vi "自动添加所有参数数据.vi"(8 "error in (no error)":errorcluster, 11 "数据类别":enum16{"水样数据", "日质控数据"}(ring)) -> (0 "错误输出":errorcluster)   [LabVIEW 2016, in "数据查询.lvlib"]
uses:
  <vilib>/Utility/config.llb/Read Key (Boolean).vi
  <vilib>/Utility/config.llb/Write Key (Boolean).vi
  <vilib>/Utility/config.llb/Read Key (String).vi
  <vilib>/Utility/config.llb/Write Key (String).vi
  <vilib>/Utility/config.llb/NI_LVConfig.lvlib
panel:
  out "数组":timestamp[](array[timestamp])
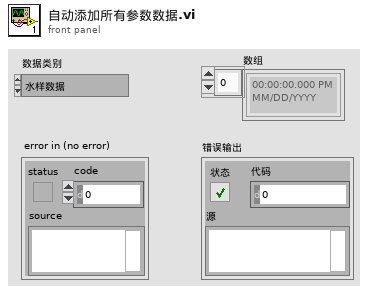
[diagram p1: front panel]
types:
  T1 = typedef "NI_LVConfig.lvlib/Config Data RefNum.ctl" = refnum<k1>
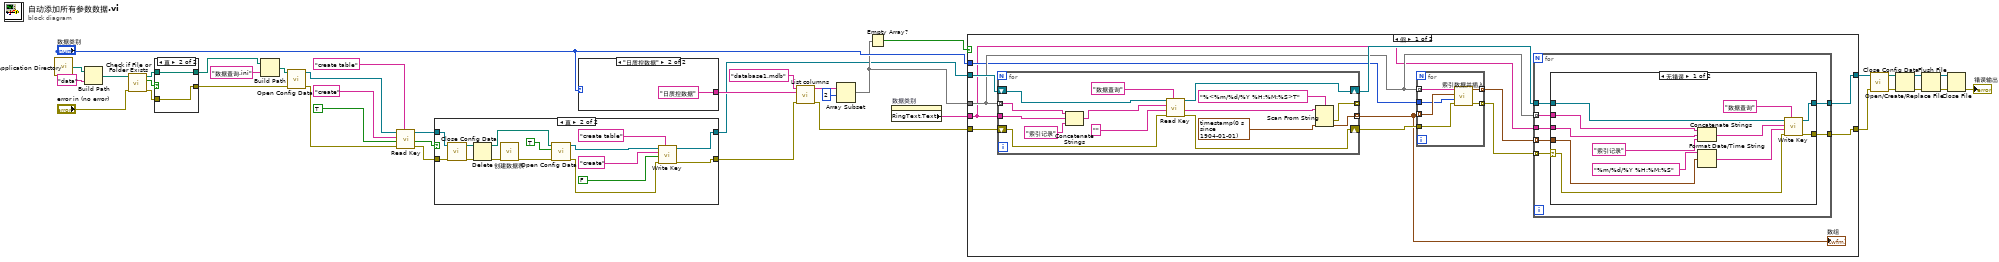
[diagram p0: block diagram]
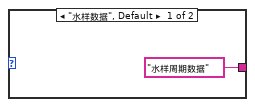
[diagram p3: hidden frame]
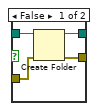
[diagram p6: hidden frame]
diagram:
  n1 = call <vilib>:"Application Directory.vi"() -> ("Application Directory"=w32:path)
  n2 = Build Path(base path=w32, name or relative path="data" ("名称或相对路径")) -> (appended path=w34:path)
  n3 = call <vilib>:"Check if File or Folder Exists.vi"("error in (no error)"="error in (no error)", "path"=w34) -> ("error out"=w37:errorcluster, "file or folder exists?"=w35:bool, "dup path"=w36:path)  [unwired: 7 in]
  n4 = case shown="真" w35 {
    tunnel: w36 -> [w43 w45]
    tunnel: w37 -> [w42 w44]
    tunnel: [w41 w45] -> w38
    tunnel: [w40 w44] -> w23
    frame False {
      n5 = Create Folder(path (use dialog)=w43, error in=w42) -> (created path=w41:path, error out=w40:errorcluster)  [unwired: 1 in, 1 out]
    }
    frame True {
    }
  }
  n6 = Build Path(base path=w38, name or relative path="数据查询.ini" ("名称或相对路径")) -> (appended path=w31:path)
  n7 = call <vilib>:"Open Config Data.vi"("error in (no error)"=w23, "configuration file path"=w31) -> ("error out"=w11:errorcluster, "refnum"=w10:T1)  [unwired: 7 in, 1 out]
  n8 = call-poly <vilib>:"Read Key.vi"("section"="create table", "error in (no error)"=w11, "default value"=TRUE, "key"="create", "refnum"=w10) -> ("error out"=w5:errorcluster, "value"=w6:bool, "refnum out"=w4:T1)  [unwired: 3 in, 1 out]
  n9 = case shown="真" w6 {
    tunnel: w5 -> [w46 w56]
    tunnel: w4 -> [w47 w62]
    tunnel: [w47 w58] -> w3
    tunnel: [w46 w57] -> w2
    frame False {
    }
    frame True {
      n10 = call <vilib>:"Close Config Data.vi"("error in (no error)"=w56, "refnum"=w62) -> ("error out"=w54:errorcluster, "file path"=w55:path)  [unwired: 8 in]
      n11 = Delete(path (use dialog)=w55, error in=w54) -> (deleted path=w52:path, error out=w53:errorcluster)  [unwired: 3 in, 1 out]
      n12 = call "创建数据表.vi"("error in (no error)"=w53) -> ("error out"=w51:errorcluster)  [unwired: 10 in]
      n13 = call <vilib>:"Open Config Data.vi"("error in (no error)"=w51, "create file if necessary (T)"=TRUE, "configuration file path"=w52) -> ("error out"=w48:errorcluster, "refnum"=w49:T1)  [unwired: 6 in, 1 out]
      n14 = call-poly <vilib>:"Write Key.vi"("section"="create table", "error in (no error)"=w48, "value"=FALSE, "key"="create", "refnum"=w49) -> ("error out"=w57:errorcluster, "refnum out"=w58:T1)  [unwired: 4 in, 1 out]
    }
  }
  n15 = case shown="\"日质控数据\"" "数据类别" {
    tunnel: ["水样周期数据" ("table") "日质控数据" ("table")] -> w15
    frame "水样数据", Default {
    }
    frame "日质控数据" {
    }
  }
  n16 = call "List columns.vi"("error in (no error)"=w2, "table"=w15, "database"="database1.mdb") -> ("error out"=w1:errorcluster, "columns"=w14:string[])  [unwired: 7 in]
  n17 = Array Subset(array=w14, index=2 ("索引")) -> (w12:string[])  [unwired: 1 in]
  n18 = Empty Array?(array=w12) -> (empty?=w22:bool)
  n19 = property on="数据类别" class="Enum (严格)"() -> ("RingText.Text"=w20:string)  [unwired: 2 in, 2 out]
  n20 = case shown="假" w22 {
    tunnel: [w75 w120] -> w25
    tunnel: [w74 w119] -> w24
    tunnel: w3 -> [w73 w120]
    tunnel: w1 -> [w72 w119]
    tunnel: w12 -> [w70 _]
    tunnel: "数据类别" -> [w67 _]
    tunnel: w20 -> [w66 _]
    frame False {
      n21 = for {
        shift-right: [w110] -> w71
        shift-left: w73 -> [w112]
        shift-right: [w109] -> w69
        shift-left: w72 -> [w111]
        tunnel: w70 -> [w101] mode=indexing
        tunnel: [w103] -> w65 mode=indexing
        tunnel: [w102] -> _ mode=indexing
        tunnel: w66 -> [w100]
        n22 = Concatenate Strings(w101, w100, "索引记录" ("key")) -> (w106:string)
        n23 = call-poly <vilib>:"Read Key.vi"("section"="数据查询", "error in (no error)"=w111, "default value"="", "key"=w106, "refnum"=w112) -> ("error out"=w109:errorcluster, "value"=w99:string, "refnum out"=w110:T1)  [unwired: 3 in, 1 out]
        n24 = Scan From String(format string="%<%m/%d/%Y %H:%M:%S>T" ("格式字符串"), input string=w99, default 1=timestamp(0 s since 1904-01-01) ("默认值 1")) -> (error out=w102:errorcluster, output 1=w103:timestamp)  [unwired: 2 in, 2 out]
      }
      "数组" <- w65
      n25 = for {
        tunnel: w65 -> [w118] mode=indexing
        tunnel: w70 -> [w117] mode=indexing
        tunnel: [w116] -> w68 mode=indexing
        tunnel: [w115] -> w76 mode=indexing
        tunnel: w69 -> [w114]
        tunnel: w67 -> [w113]
        n26 = call "索引数据并插入.vi"("error in (no error)"=w114, "数据类别"=w113, "索引记录"=w118, "table"=w117) -> ("error out"=w116:errorcluster, "最新索引记录"=w115:timestamp)  [unwired: 6 in]
      }
      n27 = for {
        tunnel: w70 -> [w83] mode=indexing
        tunnel: w76 -> [w82] mode=indexing
        tunnel: w71 -> [w81]
        tunnel: w68 -> [w78] mode=indexing
        tunnel: [w80] -> w75
        tunnel: [w79] -> w74
        tunnel: w66 -> [w77]
        n28 = case shown="无错误" w78 {
          selector: w78 -> [w86 w96]
          tunnel: w83 -> [w85 _]
          tunnel: w82 -> [w92 _]
          tunnel: w81 -> [w90 w97]
          tunnel: [w89 w97] -> w80
          tunnel: [w88 w96] -> w79
          tunnel: w77 -> [w84 _]
          frame No Error {
            n29 = Concatenate Strings(w85, w84, "索引记录" ("key")) -> (w93:string)
            n30 = Format Date/Time String(time format string (%c)="%m/%d/%Y %H:%M:%S" ("时间格式字符串(%c)"), seconds (now)=w92) -> (date/time string=w91:string)  [unwired: 1 in]
            n31 = call-poly <vilib>:"Write Key.vi"("section"="数据查询", "error in (no error)"=w86, "value"=w91, "key"=w93, "refnum"=w90) -> ("error out"=w88:errorcluster, "refnum out"=w89:T1)  [unwired: 4 in, 1 out]
          }
          frame Error {
          }
        }
      }
    }
    frame True {
    }
  }
  n32 = call <vilib>:"Close Config Data.vi"("error in (no error)"=w24, "refnum"=w25) -> ("error out"=w30:errorcluster, "file path"=w21:path)  [unwired: 8 in]
  n33 = Open/Create/Replace File(file path (use dialog)=w21, error in=w30) -> (refnum out=w26:refnum<file>, error out=w27:errorcluster)  [unwired: 4 in, 1 out]
  n34 = Flush File(refnum=w26, error in=w27) -> (refnum out=w28:refnum<file>, error out=w29:errorcluster)
  n35 = Close File(refnum=w28, error in=w29) -> (error out=→"错误输出":errorcluster)  [unwired: 1 out]
